vi "problem.vi"() -> ()   [LabVIEW 2014]
panel:
  out "Boolean":bool
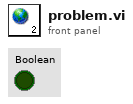
[diagram p1: front panel]
diagram:
